vi "Index Param Array.vi"(8 "Index":u8, 11 "Array Input":dbl[](array[numeric])) -> (3 "Index Output":dbl)   [LabVIEW 2016]
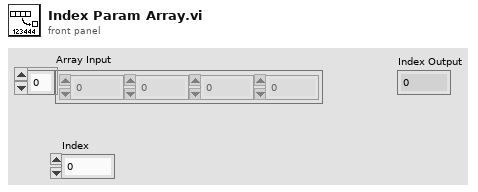
[diagram p1: front panel]
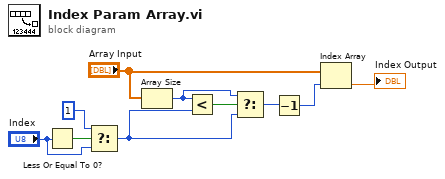
[diagram p0: block diagram]
diagram:
  n1 = Less Or Equal To 0?(x="Index") -> (x <= 0?=w4:bool)
  n2 = Select(t=1 ("size(s)"), s=w4, f="Index") -> (s? t:f=w3:i32)
  n3 = Array Size(array="Array Input") -> (size(s)=w8:i32)
  n4 = Less?(x=w8, y=w3) -> (x < y?=w9:bool)
  n5 = Select(t=w8, s=w9, f=w3) -> (s? t:f=w7:i32)
  n6 = Decrement(x=w7) -> (x-1=w6:i32)
  n7 = Index Array(array="Array Input", index=w6) -> (element=→"Index Output":dbl)
